vi "Versus.vi"(11 "DataIn":T1) -> (3 "DataOut":T1)   [LabVIEW 2017]
doc: "SubVI criada para apagar a coluna de adversário na linha de quem convidou e de quem foi convidado no caso de recusa ou de fim de jogo"
uses:
  controls/DataIn.ctl
  controls/Tabuleiro.ctl
  controls/GameOption.ctl
  controls/Table.ctl
  <vilib>/Utility/file.llb/Write Delimited Spreadsheet (string).vi
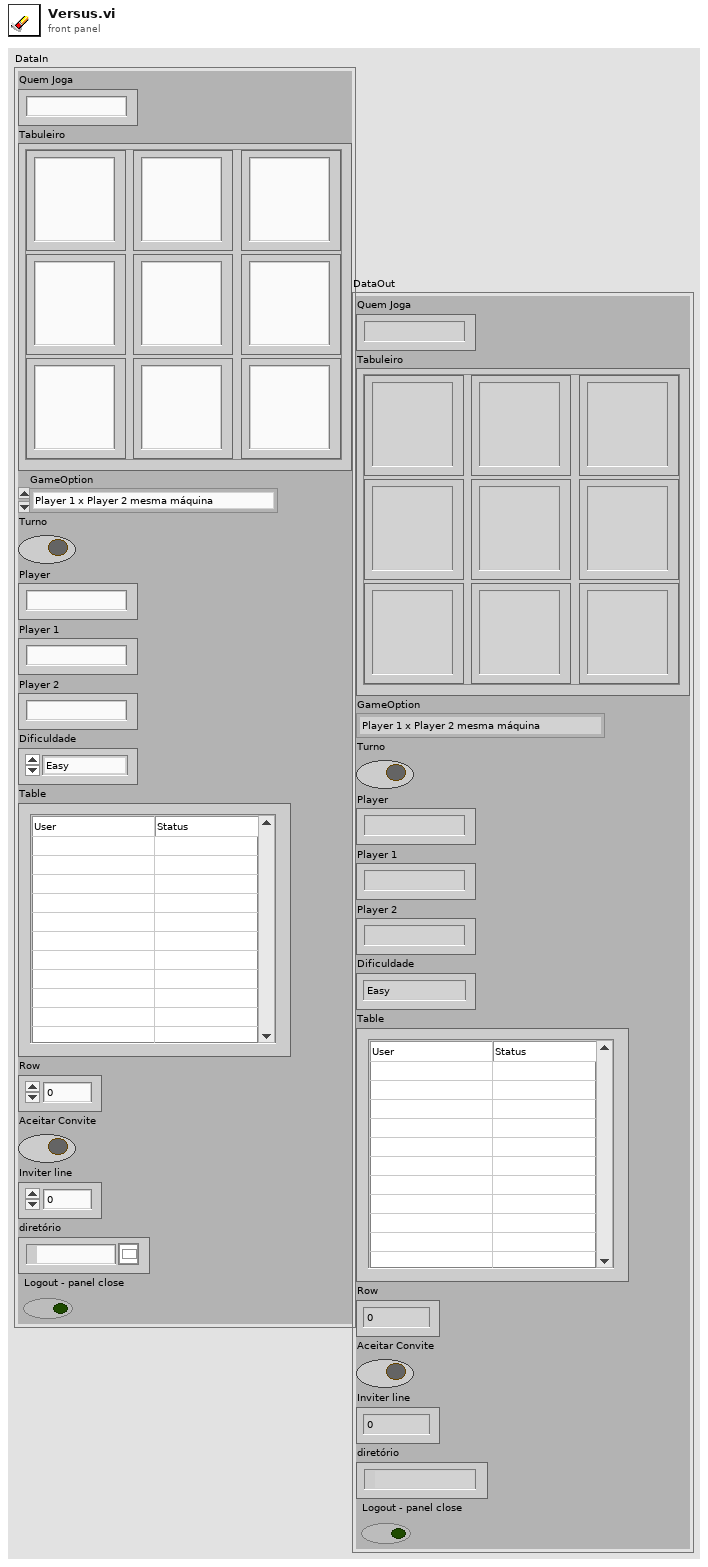
[diagram p1: front panel]
types:
  T1 = typedef "DataIn.ctl" = cluster{"Quem Joga":string, "Tabuleiro":T2, "GameOption":T3, "Turno":bool, "Player":string, "Player 1":string, "Player 2":string, "Dificuldade":enum16{"Easy", "Medium", "Hard"}, "Table":T4, "Row":u32, "Aceitar Convite":bool, "Inviter line":u32, "diretório":path, "Logout - panel close":bool}
  T2 = typedef "Tabuleiro.ctl" = cluster{"(0,0)":string, "(1,0)":string, "(0,1)":string, "(1,1)":string, "(2,0)":string, "(1,2)":string, "(2,2)":string, "(0,2)":string, "(2,1) ":string}
  T3 = typedef "GameOption.ctl" = enum16{"Player 1 x Player 2 mesma máquina", "Player 1 x Player 2 pela rede", "Player 1 x Computador", "Wait for Event", "Initialize", "Stop"}
  T4 = typedef "Table.ctl" = string[][]
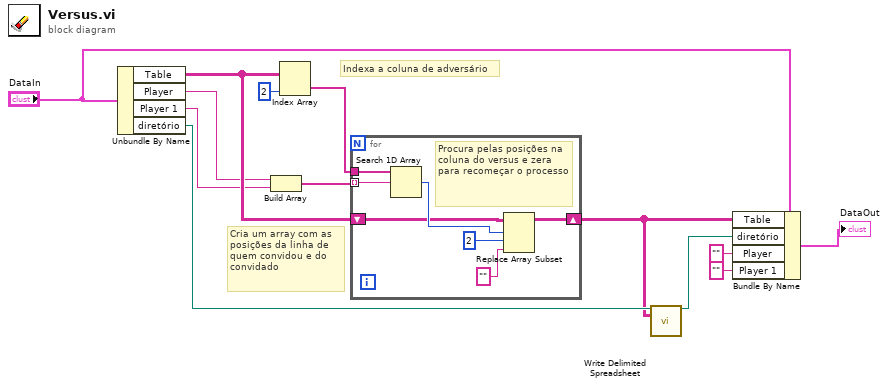
[diagram p0: block diagram]
diagram:
  # "Cria um array com as posições da linha de quem convidou e do convidado"
  # "Indexa a coluna de adversário"
  n1 = Unbundle By Name("DataIn") -> ("Table"=w9:T4, "Player"=w7:string, "Player 1"=w6:string, "diretório"=w5:path)
  n2 = Build Array(w7, w6) -> (w8:string[])
  n3 = Index Array(array=w9, index (col)=2 ("disabled index (col)")) -> (element=w11:string[])  [unwired: 1 in]
  n4 = for {
    tunnel: w8 -> [w14] mode=indexing
    tunnel: w11 -> [w17]
    shift-right: [w15] -> w3
    shift-left: w9 -> [w16]
    # "Procura pelas posições na coluna do versus e zera para recomeçar o processo"
    n5 = Search 1D Array(1D array=w17, element=w14) -> (index of element=w18:i32)  [unwired: 1 in]
    n6 = Replace Array Subset(array=w16, new element="", index (row)=w18, index (col)=2 ("disabled index (col)")) -> (w15:T4)
  }
  n7 = call-poly <vilib>:"Write Delimited Spreadsheet.vi"("file path (dialog if empty)"=w5, "2D data"=w3) -> ("new file path (Not A Path if cancelled)"=w4:path)  [unwired: 12 in, 1 out]
  n8 = Bundle By Name(cluster="DataIn", "Table"=w3, "diretório"=w4, "Player"="", "Player 1"="") -> (→"DataOut":T1)
